vi "Maui.Config.Read.vi"(8 "error in (no error)":errorcluster, 10 "INI Fomatted Cluster Type":variant, 11 "Maui.Config in":refnum<class "Maui.Config.lvclass">) -> (0 "error out":errorcluster, 2 "INI Fomatted Cluster":variant, 3 "Maui.Config out":refnum<class "Maui.Config.lvclass">)   [LabVIEW 2020, in "Maui.Config.lvclass"]
uses:
  Maui.Config.lvclass
  <vilib>/Utility/config.llb/NI_LVConfig.lvlib
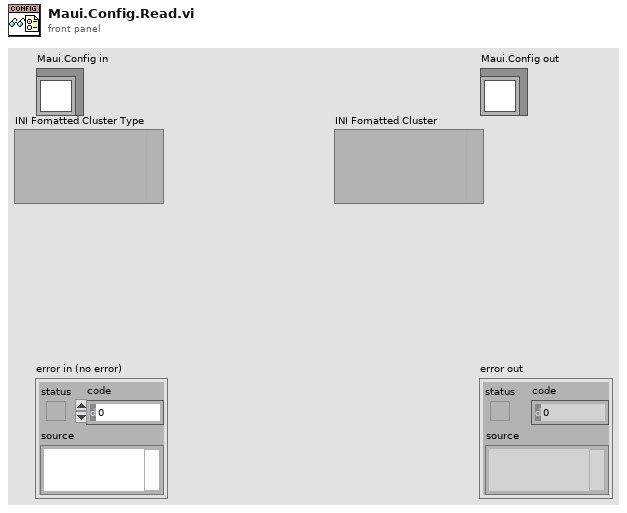
[diagram p1: front panel]
types:
  T1 = typedef "NI_LVConfig.lvlib/Config Data RefNum.ctl" = refnum<k1>
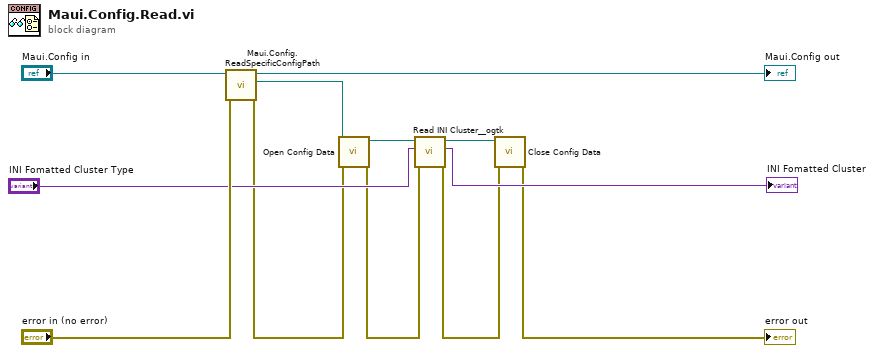
[diagram p0: block diagram]
diagram:
  n1 = call "Maui.Config.ReadSpecificConfigPath.vi"("error in (no error)"="error in (no error)", "Maui.Config in"="Maui.Config in") -> ("error out"=w3:errorcluster, "Specific Configuration"=w1:path, "Maui.Config out"=→"Maui.Config out":refnum<class "Maui.Config.lvclass">)  [unwired: 7 in]
  n2 = call <vilib>:"Open Config Data.vi"("error in (no error)"=w3, "configuration file path"=w1) -> ("error out"=w6:errorcluster, "refnum"=w7:T1)  [unwired: 7 in, 1 out]
  n3 = call <userlib>:"Read INI Cluster__ogtk.vi"("error in (no error)"=w6, "INI Fomatted Cluster Type"="INI Fomatted Cluster Type", "refnum"=w7) -> ("error out"=w4:errorcluster, "INI Fomatted Cluster"=→"INI Fomatted Cluster":variant, "dup refnum"=w5:T1)  [unwired: 4 in, 2 out]
  n4 = call <vilib>:"Close Config Data.vi"("error in (no error)"=w4, "refnum"=w5) -> ("error out"=→"error out":errorcluster)  [unwired: 8 in, 1 out]
